vi "Update Led.vi"(8 "error in":errorcluster, 9 "color":T1, 10 "light on":bool, 11 "led":refnum<vi>) -> (0 "error out":errorcluster, 1 "color":T1, 2 "light on out":bool, 3 "led out":refnum<vi>)   [LabVIEW 2010, in "Twinkle Button.xctl"]
doc: "本VI是为《我和LabVIEW》一书编写的示例。\n关于本书的介绍请参考网页：\nhttp://ruanqizhen.spaces.live.com/blog/cns!5852D4F797C53FB6!4310.entry"
uses:
  Twinkle Button.xctl
  Data.ctl
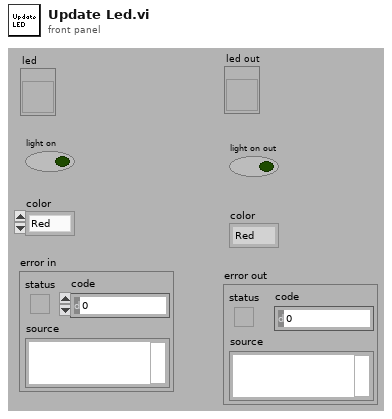
[diagram p1: front panel]
types:
  T1 = typedef "Twinkle Button.xctl/Data.ctl" = enum16{"Red", "Green", "Blue"}
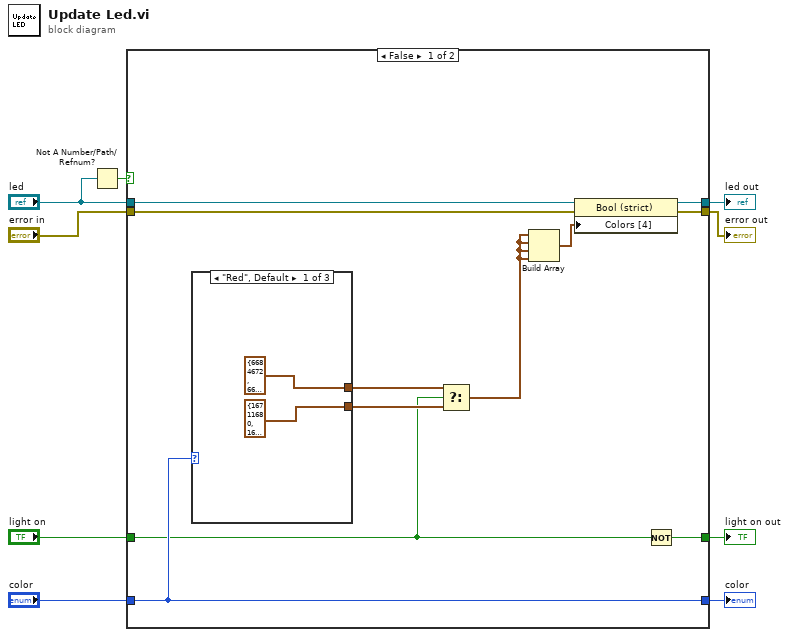
[diagram p0: block diagram]
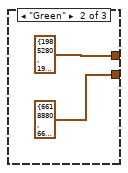
[diagram p2: hidden frame]
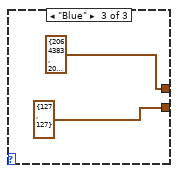
[diagram p3: hidden frame]
diagram:
  n1 = Not A Number/Path/Refnum?(number/path/refnum="led") -> (NaN/Path/Refnum?=w6:bool)
  n2 = case shown="False" w6 {
    tunnel: "light on" -> [w11 w29]
    tunnel: "led" -> [w19 w30]
    tunnel: "error in" -> [w18 w27]
    tunnel: [w17 w27] -> w3
    tunnel: [w16 w30] -> w4
    tunnel: "color" -> [w14 w28]
    tunnel: [w15 w29] -> w8
    tunnel: [w14 w28] -> w9
    frame False {
      n3 = case shown="\"Red\", Default" w14 {
        tunnel: [cluster{u32, u32} {6684672, 6684672} cluster{u32, u32} {1985280, 1985280} cluster{u32, u32} {2064383, 2064383}] -> w13
        tunnel: [cluster{u32, u32} {16711680, 16711680} cluster{u32, u32} {6618880, 6618880} cluster{u32, u32} {127, 127}] -> w12
        frame "Red", Default {
        }
        frame "Green" {
        }
        frame "Blue" {
        }
      }
      n4 = Select(t=w13, s=w11, f=w12) -> (s? t:f=w10:cluster{u32, u32})
      n5 = Build Array(w10, w10, w10, w10) -> (w20:cluster{u32, u32}[])
      n6 = property class="Bool (strict)"(reference=w19, error in=w18, "Colors [4]"=w20) -> (reference out=w16:refnum<vi>, error out=w17:errorcluster)
      n7 = Not(x=w11) -> (.not. x?=w15:bool)
    }
    frame True {
    }
  }
  "color" <- w9
  "light on out" <- w8
  "led out" <- w4
  "error out" <- w3
